vi "moveToPosition.vi"(0 "MultiAxisController in":refnum<class "_MultiAxisController.lvclass">, 2 "target(s) (in)":T1[](array[typedef]), 5 "error in (no error)":errorcluster) -> (14 "MultiAxisController out":refnum<class "_MultiAxisController.lvclass">, 17 "success?":bool, 18 "response":string, 19 "error out":errorcluster)   [LabVIEW 2020, in "classes.lvlib" / "_MultiAxisController.lvclass"]
doc: "Produced By:\n\n<B>Kod Integrations, LLC</B>\n4835 Marianne Drive\nMount Airy, MD 21771\nhttp://www.kodintegrations.com\nemail: info@kodintegrations.com\nphone: (240) 687-1288"
uses:
  _MultiAxisController.lvclass
  _Controller.lvclass
  C:/GEECS/Developers Version/source/Device Drivers/Newmark-NSC-A/Arcus Driver 3.0.0/ArcusUsbComm/classes/Controller/_Controller.lvclass
  C:/GEECS/Developers Version/source/Device Drivers/Newmark-NSC-A/Arcus Driver 3.0.0/ArcusUsbComm/classes/MultiAxisController/_MultiAxisController.lvclass
  axis.ctl
  common.lvlib
  movement_item.ctl
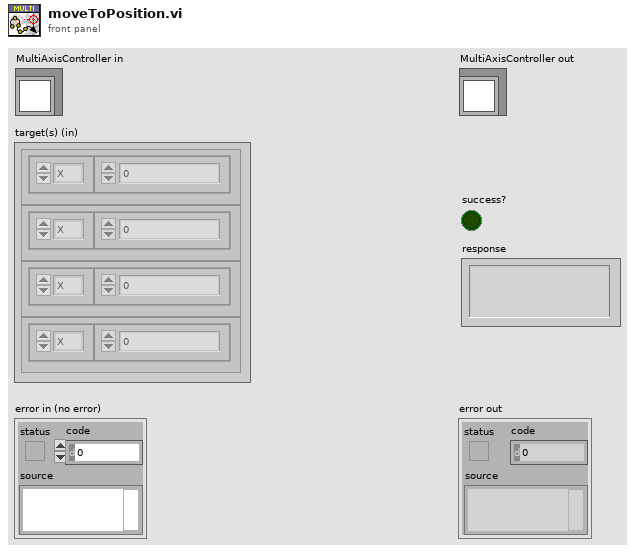
[diagram p1: front panel]
types:
  T1 = typedef "common.lvlib/movement_item.ctl" = cluster{"axis":T2, "target":i32}
  T2 = typedef "common.lvlib/axis.ctl" = enum16{"X", "Y", "Z", "U"}
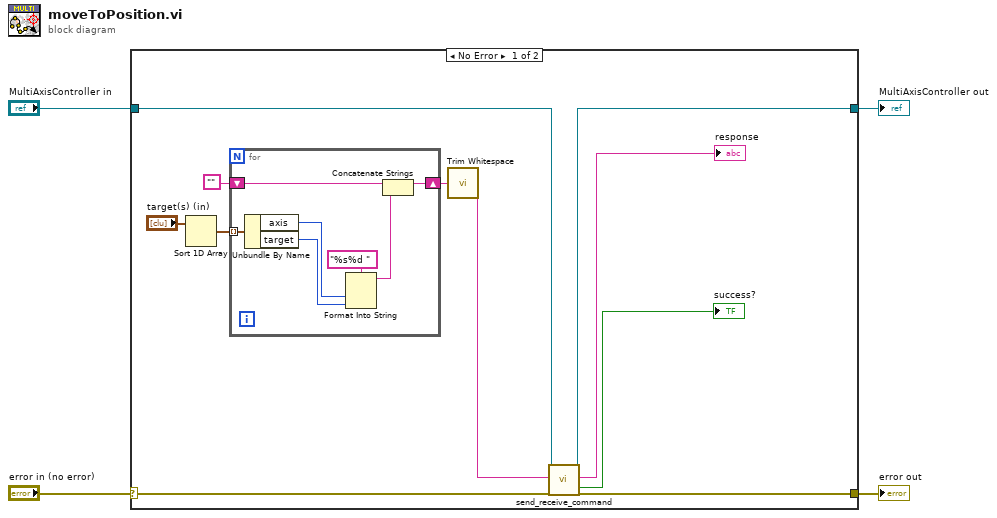
[diagram p0: block diagram]
diagram:
  n1 = case shown="No Error" "error in (no error)" {
    selector: "error in (no error)" -> [w15 w24]
    tunnel: [w14 w24] -> w3
    tunnel: [w12 w23] -> w1
    tunnel: "MultiAxisController in" -> [w13 w23]
    frame No Error {
      n2 = Sort 1D Array(array="target(s) (in)") -> (sorted array=w8:T1[])
      n3 = for {
        tunnel: w8 -> [w21] mode=indexing
        shift-right: [w16] -> w6
        shift-left: "" -> [w18]
        n4 = Unbundle By Name(w21) -> ("axis"=w20:T2, "target"=w19:i32)
        n5 = Format Into String(format string="%s%d ", w20, w19) -> (resulting string=w17:string)  [unwired: 2 in, 1 out]
        n6 = Concatenate Strings(w18, w17) -> (w16:string)
      }
      n7 = call "Trim Whitespace.vi"("string"=w6) -> ("trimmed string"=w5:string)  [unwired: 1 in]
      n8 = call "send_receive_command.vi"("reference (in)"=w13, "ASCII Command (in)"=w5, "error in (no error)"=w15) -> ("reference (out)"=w12:refnum<class "_MultiAxisController.lvclass">, "response (out)"=→"response":string, "success?"=→"success?":bool, "error out"=w14:errorcluster)  [unwired: 12 in, 1 out]
    }
    frame Error {
    }
  }
  "error out" <- w3
  "MultiAxisController out" <- w1
